vi "IsDataSetMsg.vi"(10 "MessageName":string) -> (2 "IsDataSet":bool)   [LabVIEW 2017, in "MessageGen.lvlib"]
uses:
  <vilib>/addons/InsightCM/MessageBus/CodeGen/MessageGen.lvlib
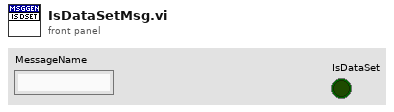
[diagram p1: front panel]
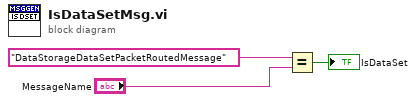
[diagram p0: block diagram]
diagram:
  n1 = Equal?(x="DataStorageDataSetPacketRoutedMessage" ("name or relative path"), y="MessageName") -> (x = y?=→"IsDataSet":bool)
